vi "Set Limits.vi"(0 "object in":refnum<class "HPS-17000-PowerModule.lvclass">, 5 "limits":T1, 11 "Error In":errorcluster) -> (4 "object out":refnum<class "HPS-17000-PowerModule.lvclass">, 15 "Error Out":errorcluster)   [LabVIEW 2023, in "HPS-17000-PowerModule.lvlib" / "HPS-17000-PowerModule.lvclass"]
uses:
  HPS-17000-PowerModule.lvclass
  builds/PowerModuleInterface/home/lvuser/natinst/bin/PowerModuleInterface.lvlibp/Classes/PowerModule_interface/Limits.ctl
  <instrlib>/HPS-17000/Client Facing Datatypes/Limits.ctl
  <instrlib>/HPS-17000/Internal/Set Limits Multi.vi
  <instrlib>/HPS-17000/HPS-17000.lvclass
  builds/PowerModuleInterface/home/lvuser/natinst/bin/PowerModuleInterface.lvlibp/Classes/PowerModule_interface/PowerModuleInterface.lvclass
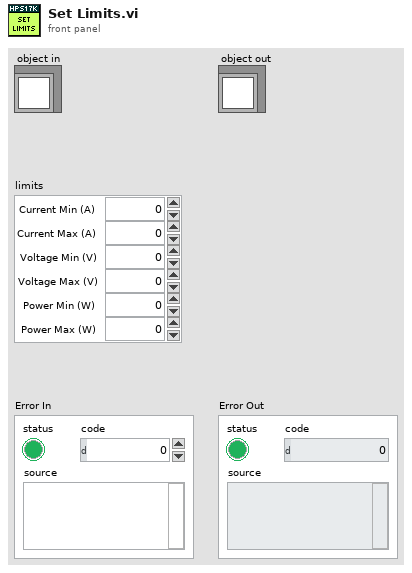
[diagram p1: front panel]
types:
  T1 = typedef "PowerModuleInterface.lvlibp/PowerModuleInterface.lvclass/Limits.ctl" = cluster{"Current Max (A)":dbl, "Current Min (A)":dbl, "Voltage Max (V)":dbl, "Voltage Min (V)":dbl, "Power Max (W)":dbl, "Power Min (W)":dbl}
  T2 = typedef "HPS-17000.lvclass/Limits.ctl" = cluster{"Current Max Limit":sgl, "Current Min Limit":sgl, "Voltage Max Limit":sgl, "Voltage Min Limit":sgl, "Power Max Limit":sgl, "Power Min Limit":sgl}
  T3 = typedef "HPS-17000-PowerModule.lvlib/HPS-17000-PowerModule.lvclass/ObjectAttributes.ctl" = cluster{"JSON Config Path":path, "Configuration":T4, "GM ID":string, "HPS17000 Refs":refnum<class "HPS-17000.lvclass">[], "connected":bool, "reserved":bool, "events":T6, "nibatterycycler_grpc_Setpoint":T7, "last timestamp":i64, "mode":T8, "range":T9, "measurement array":T10[]}
  T4 = typedef "HPS-17000-PowerModule.lvlib/HPS-17000-PowerModule.lvclass/Configuration.ctl" = cluster{"TSN NIC IP Address":string, "HPS17000 IP Addresses":string[], "HPS Topology":enum16{"SINGLE", "MULTI"}, "Setpoint Stream Config":T5, "Measurement Array Size":i32}
  T5 = typedef "Cycler.lvclass/Setpoint Stream Basic Config.ctl" = cluster{"local address":string, "receiver port":u16}
  T6 = typedef "HPS-17000.lvclass/Multi-Cycler Events.ctl" = cluster{"heartbeats events":refnum<user-event>[], "faults events":refnum<user-event>[], "network sync event":refnum<user-event>[], "setpoint status event":refnum<user-event>[]}
  T7 = typedef "NI_BC_client.lvlib/nibatterycycler_grpc_Setpoint.ctl" = cluster{"voltage":sgl, "current":sgl, "min_power":sgl, "max_power":sgl, "resistance":sgl}
  T8 = typedef "HPS-17000-PowerModule.lvlib/HPS-17000-PowerModule.lvclass/Mode.ctl" = u16
  T9 = typedef "PowerModuleInterface.lvlibp/PowerModuleInterface.lvclass/Range.ctl" = cluster{"Current Max (A)":dbl, "Current Min (A)":dbl, "Voltage Max (V)":dbl, "Voltage Min (V)":dbl}
  T10 = typedef "PowerModuleInterface.lvlibp/PowerModuleInterface.lvclass/Measurements.ctl" = cluster{"measured voltage (V)":dbl, "measured current (A)":dbl, "setpoint voltage (V)":dbl, "setpoint current (A)":dbl, "timestamp":dbl}
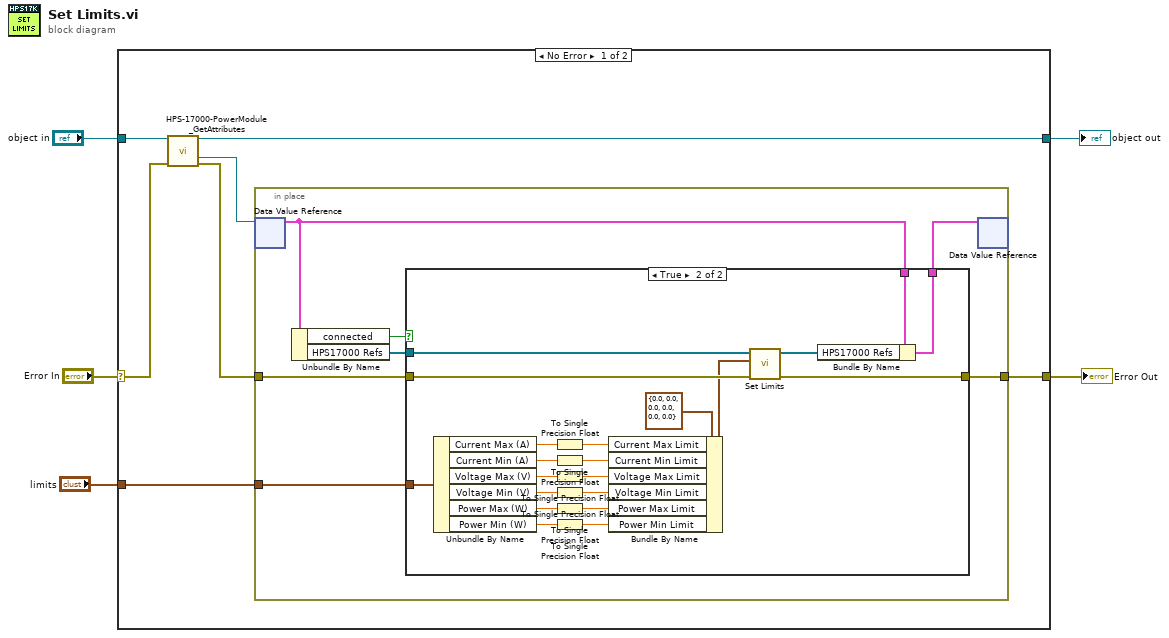
[diagram p0: block diagram]
diagram:
  n1 = case shown="No Error" "Error In" {
    selector: "Error In" -> [w12 w44]
    tunnel: [w8 w43] -> w5
    tunnel: [w9 w44] -> w3
    tunnel: "object in" -> [w7 w43]
    tunnel: "limits" -> [w6 _]
    frame No Error {
      n2 = call "HPS-17000-PowerModule_GetAttributes.vi"("reference in"=w7, "Error In"=w12) -> ("reference out"=w8:refnum<class "HPS-17000-PowerModule.lvclass">, "DataRef"=w11:refnum<data-value>, "Error Out"=w10:errorcluster)  [unwired: 10 in, 1 out]
      n3 = in-place {
        in-place-border: w10 -> [w17]
        in-place-border: [w16] -> w9
        in-place-border: w6 -> [w13]
        n4 = in-place-dvr #1(w11) -> (w18:T3)  [unwired: 1 out]
        n5 = Unbundle By Name(w18) -> ("connected"=w14:bool, "HPS17000 Refs"=w15:refnum<class "HPS-17000.lvclass">[])
        n6 = case shown="True" w14 {
          tunnel: [w21 w42] -> w19
          tunnel: w18 -> [w21 w41]
          tunnel: w17 -> [w20 w38]
          tunnel: [w20 w37] -> w16
          tunnel: w15 -> [_ w40]
          tunnel: w13 -> [_ w35]
          frame False {
          }
          frame True {
            n7 = Unbundle By Name(w35) -> ("Current Max (A)"=w33:dbl, "Current Min (A)"=w31:dbl, "Voltage Max (V)"=w29:dbl, "Voltage Min (V)"=w27:dbl, "Power Max (W)"=w25:dbl, "Power Min (W)"=w24:dbl)
            n8 = To Single Precision Float(number=w33) -> (single precision float=w32:sgl)
            n9 = To Single Precision Float(number=w31) -> (single precision float=w30:sgl)
            n10 = To Single Precision Float(number=w29) -> (single precision float=w28:sgl)
            n11 = To Single Precision Float(number=w27) -> (single precision float=w26:sgl)
            n12 = To Single Precision Float(number=w25) -> (single precision float=w22:sgl)
            n13 = To Single Precision Float(number=w24) -> (single precision float=w23:sgl)
            n14 = Bundle By Name(cluster=T2 {"Current Max Limit"=0.0, "Current Min Limit"=0.0, "Voltage Max Limit"=0.0, "Voltage Min Limit"=0.0, "Power Max Limit"=0.0, "Power Min Limit"=0.0} ("limits"), "Current Max Limit"=w32, "Current Min Limit"=w30, "Voltage Max Limit"=w28, "Voltage Min Limit"=w26, "Power Max Limit"=w22, "Power Min Limit"=w23) -> (w34:T2)
            n15 = call-poly <instrlib>:"Set Limits.vi"("error in"=w38, "limits"=w34, "cycler refs in"=w40) -> ("error out"=w37:errorcluster, "cycler refs out"=w39:refnum<class "HPS-17000.lvclass">[])  [unwired: 7 in]
            n16 = Bundle By Name(cluster=w41, "HPS17000 Refs"=w39) -> (w42:T3)
          }
        }
        n17 = in-place-dvr #1(w19) -> ()  [unwired: 2 out]
      }
    }
    frame Error {
    }
  }
  "Error Out" <- w3
  "object out" <- w5
